vi "AlGaInPAs_prep_run_cont_dil_v00.vi"(2 "Debug Mode":bool, 3 "Elapsed Time(s)":dbl, 4 "State":enum16{"Edit", "Start", "Run", "End", "Idle"}(ring), 5 "Argument List In":string[](array[string])) -> (0 "Status Out":string, 1 "Argument List Out":string[](array[string]))   [LabVIEW 2011]
panel:
  in  "Prep Al":bool caption="Pre-run"
  in  "Run Al":bool caption="Run"
  in  "Al Flow":dbl caption="Al Flow (0-100 sscm)" format="%.2f"
  in  "Ga Tab":enum32{"Page 1", "Page 2"}(tab)
  in  "Prep Ga":bool caption="Pre-run"
  in  "Run Ga":bool caption="Run"
  in  "Ga Flow":dbl caption="Ga Flow (0-100 sscm)" format="%.2f"
  in  "Dilute Ga":bool caption="Dilute"
  in  "GAMFC3":dbl caption="GAMFC3 (0-1000 sccm)"
  out "GAMFC2 set":dbl caption="GAMFC2 (0-100 sscm)" format="%.1f"
  out "GAMFC1 set":dbl caption="GAMFC1 set (0-10 sccm)"
  in  "GAMFC1":dbl caption="GAMFC1 (0-10 sscm)" format="%.2f"
  out "first":bool=TRUE
  out "total time":dbl
  out "is OK?":bool
  out "AsH3?":bool
  out "PH3?":bool
  out "In?":bool
  out "Ga?":bool
  out "Al?":bool
  in  "Prep As":bool caption="Pre-run"
  in  "Prep P":bool caption="Pre-run"
  in  "Prep In":bool caption="Pre-run"
  in  "prep_time":dbl caption="pre-run time (s)"
  in  "Run As":bool caption="Run"
  in  "AsH3 Flow":dbl caption="As Flow (0-10 sccm)" format="%.2f"
  in  "P Flow":dbl caption="P Flow (0-100 sccm)" format="%.2f"
  in  "Run P":bool caption="Run"
  in  "In Flow":dbl caption="In Flow (0-100 sscm)" format="%.2f"
  in  "Run In":bool caption="Run"
  in  "Cancel":bool
  in  "OK":bool
  out "tTotal(s) 2":dbl
  # "Add pre-run time to run time in editor."
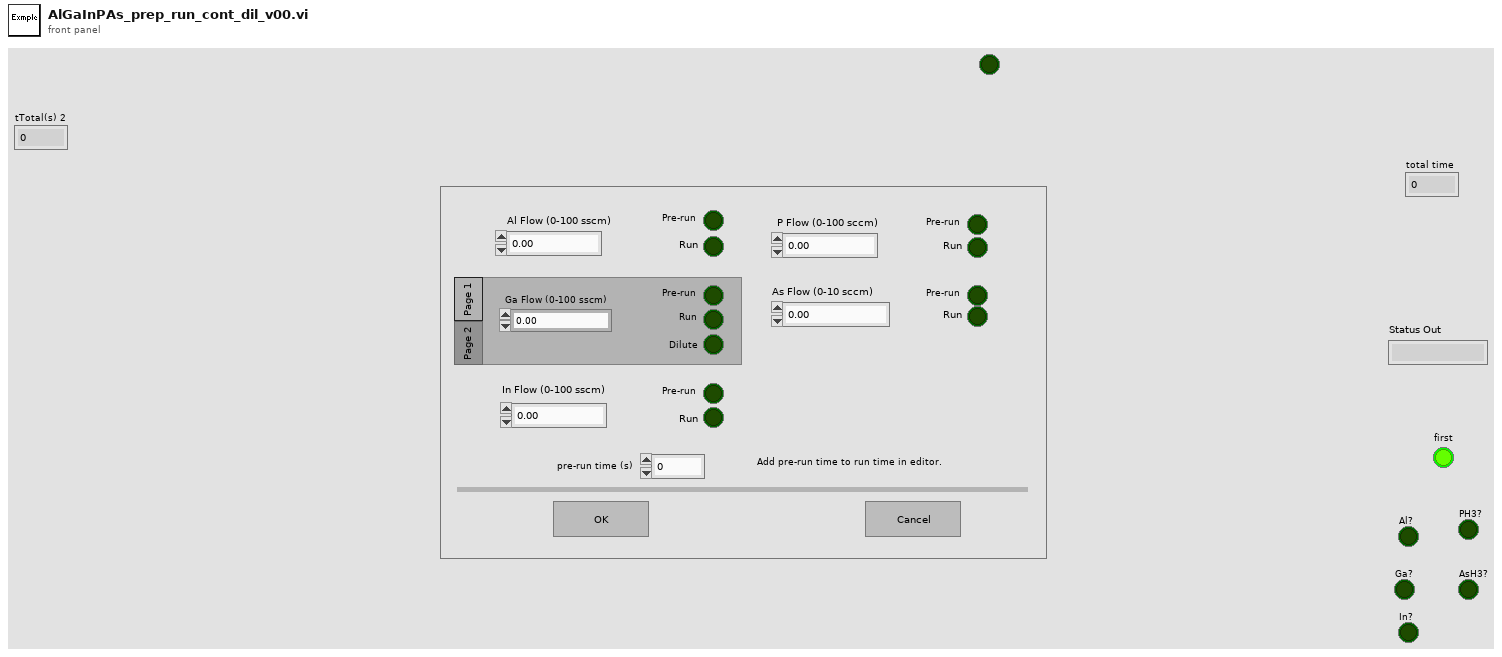
[diagram p1: front panel]
types:
  T1 = enum16{"Discrete", "Continuous", "Instantaneous"}
  T2 = enum32{"Invalid", "Default", "Floating", "Floating/Auto-Hide", "Modal"}
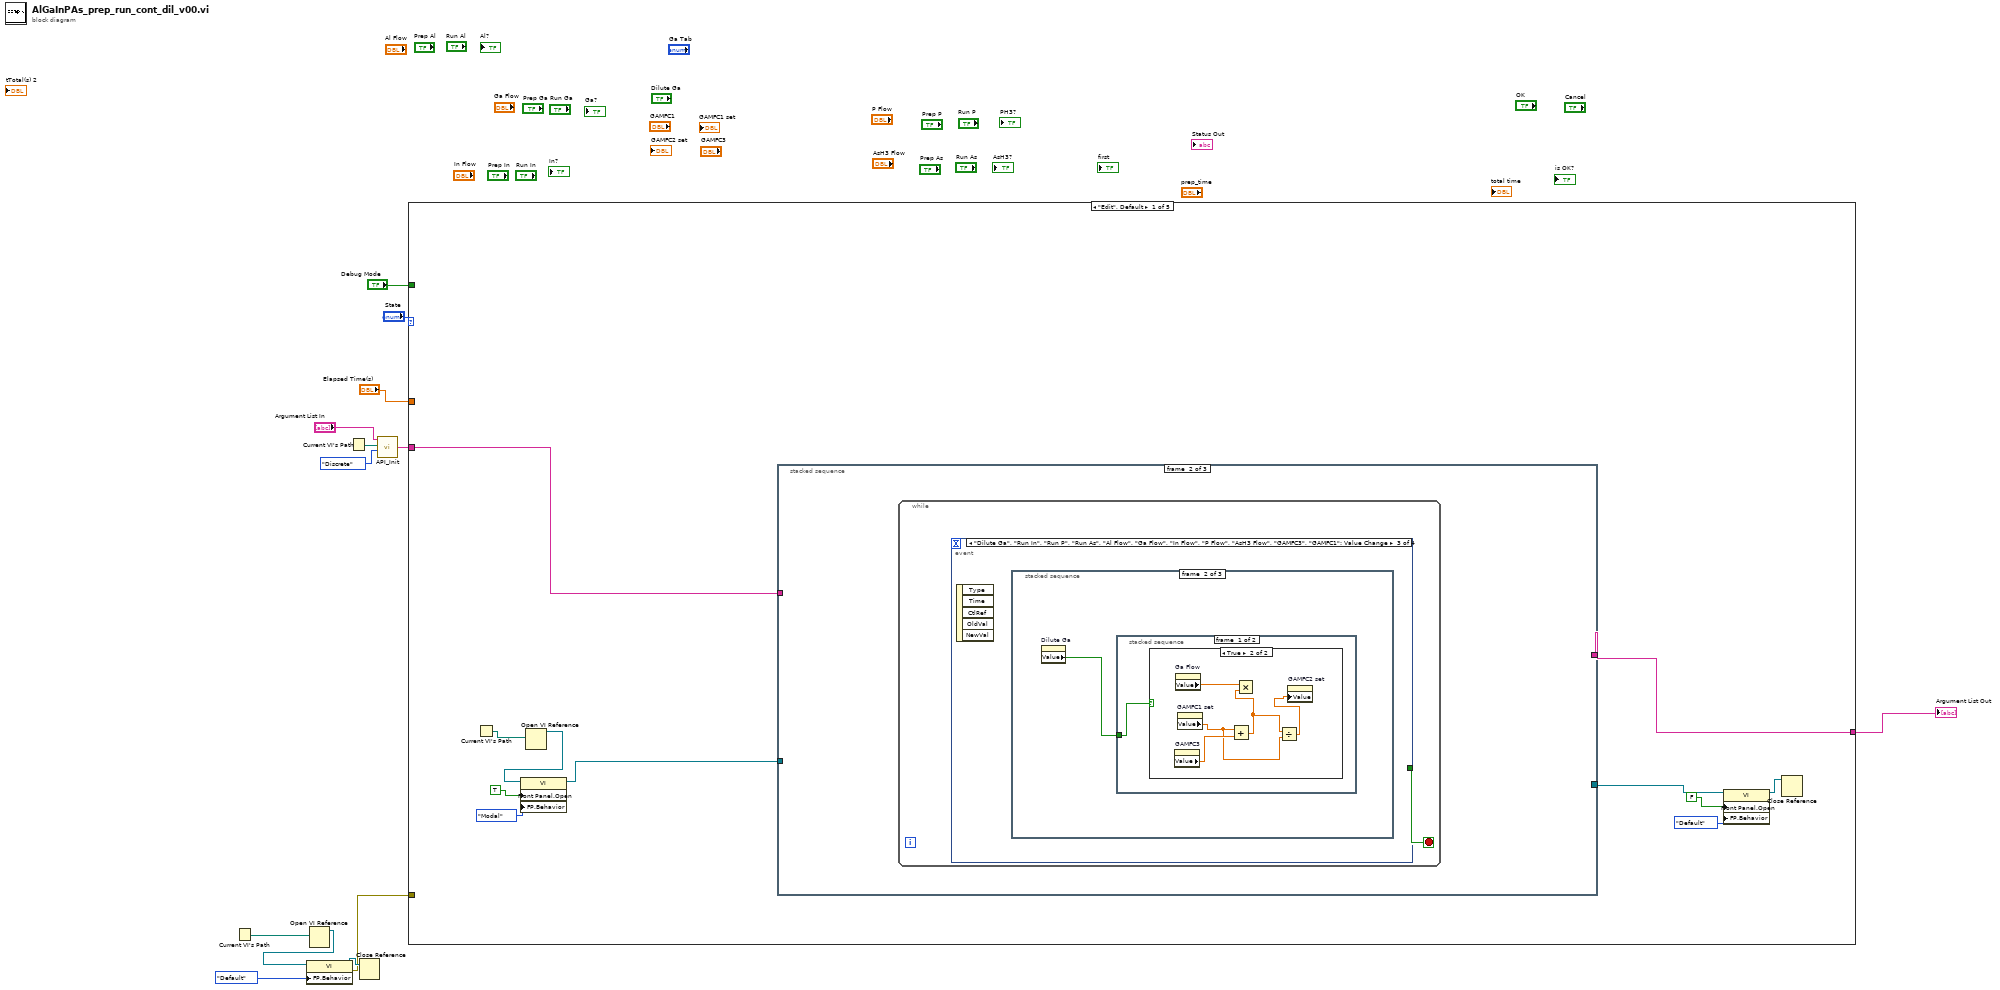
[diagram p0: block diagram]
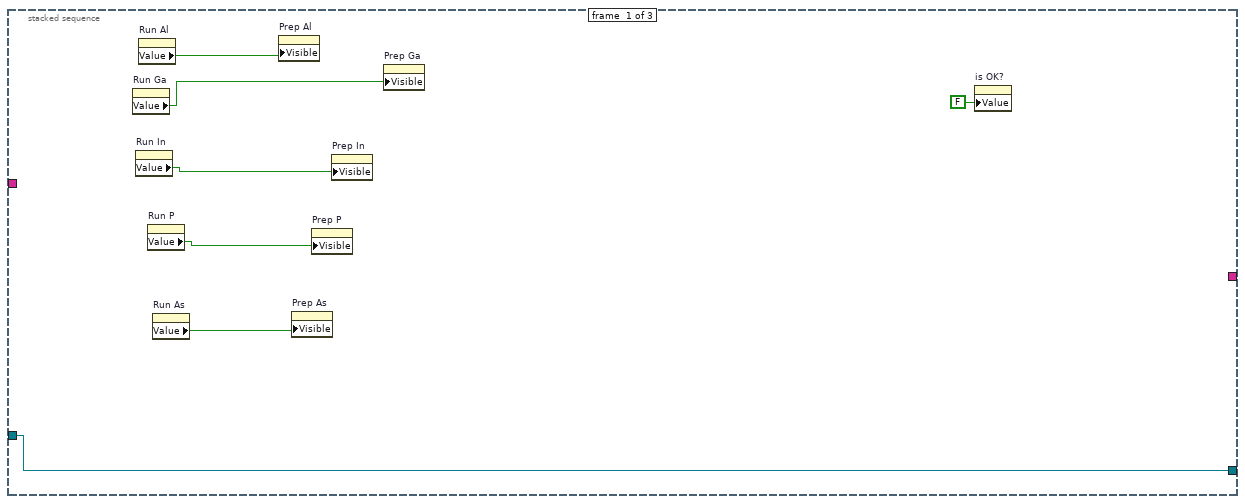
[diagram p2: hidden frame]
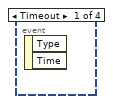
[diagram p3: hidden frame]
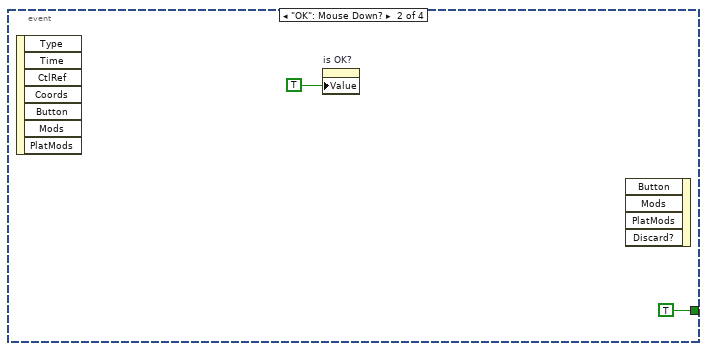
[diagram p4: hidden frame]
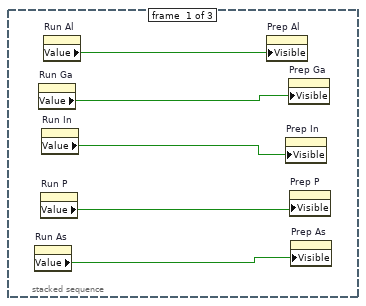
[diagram p5: hidden frame]
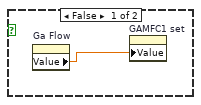
[diagram p6: hidden frame]
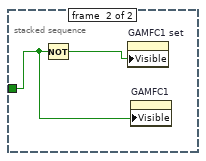
[diagram p7: hidden frame]
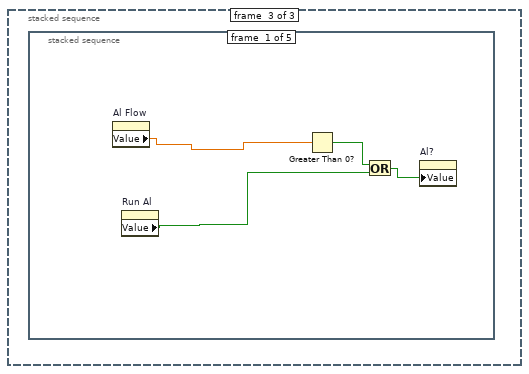
[diagram p8: hidden frame]
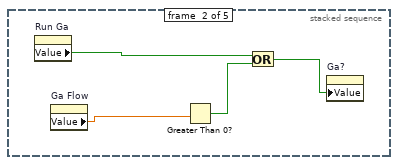
[diagram p9: hidden frame]
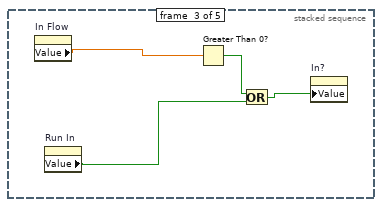
[diagram p10: hidden frame]
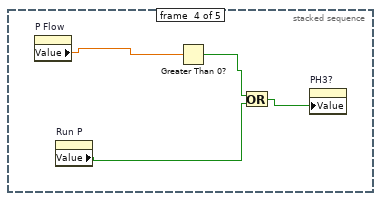
[diagram p11: hidden frame]
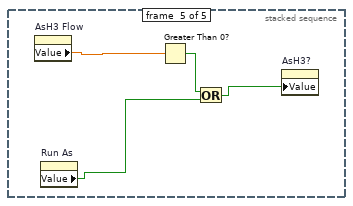
[diagram p12: hidden frame]
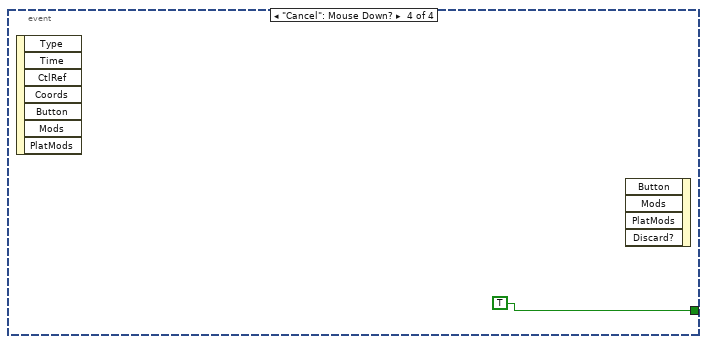
[diagram p13: hidden frame]
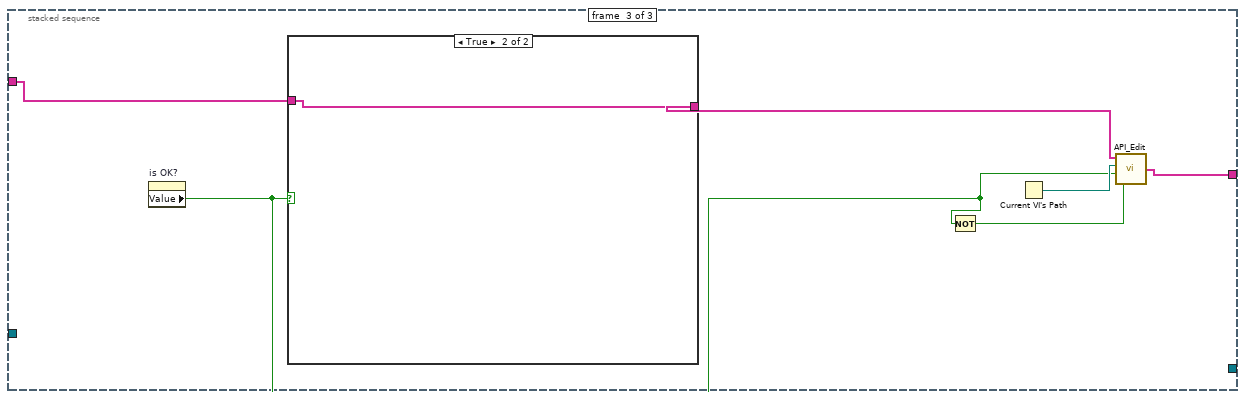
[diagram p14: hidden frame]
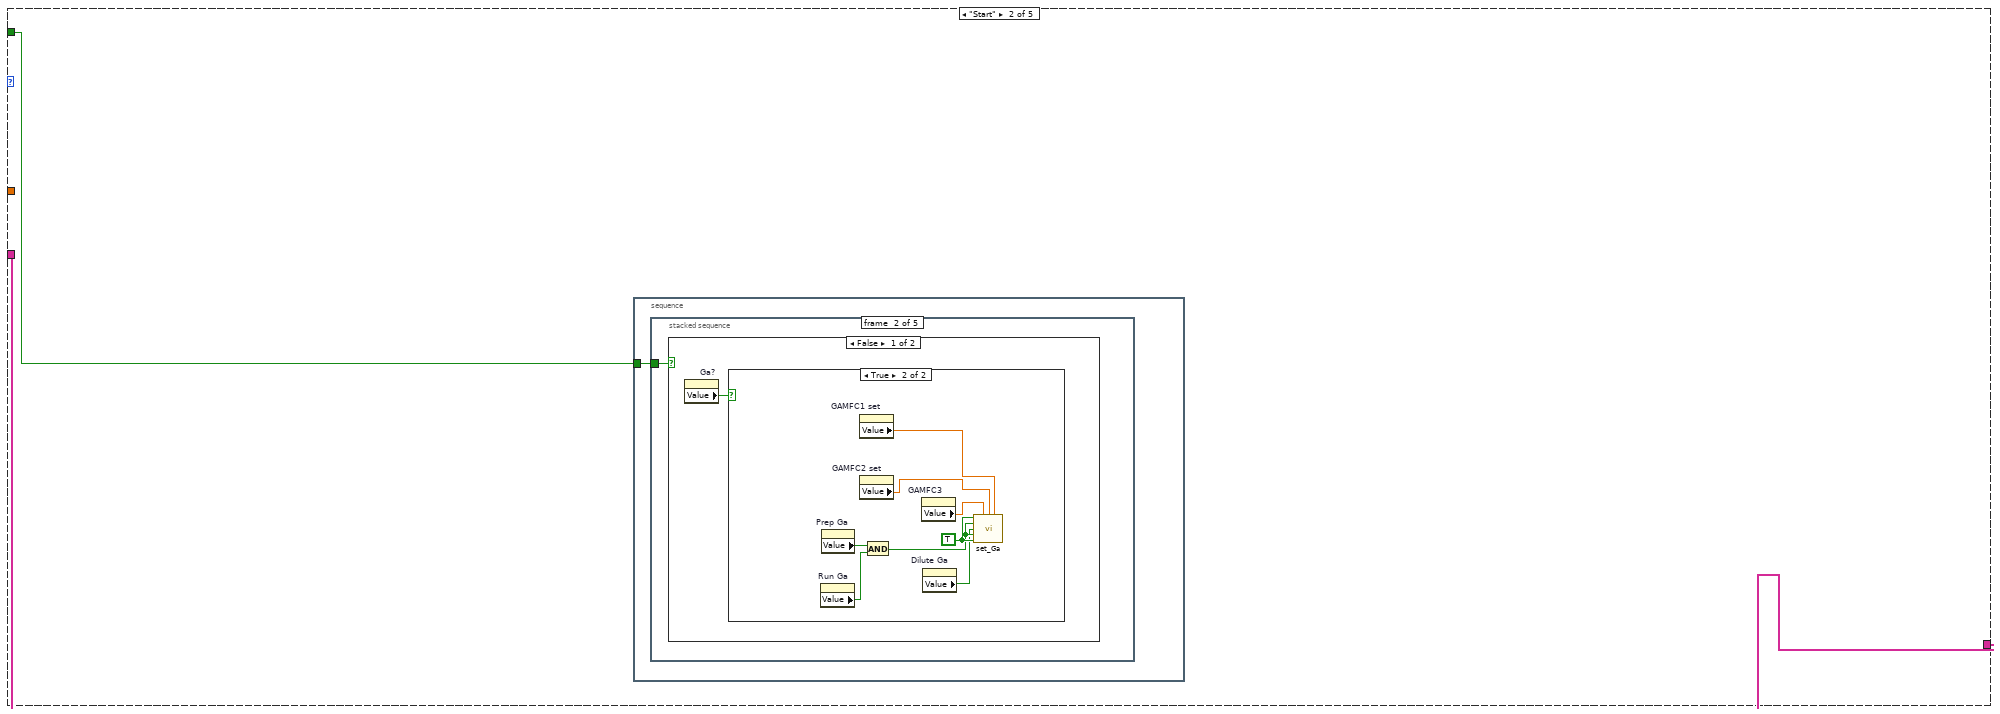
[diagram p16: hidden frame]
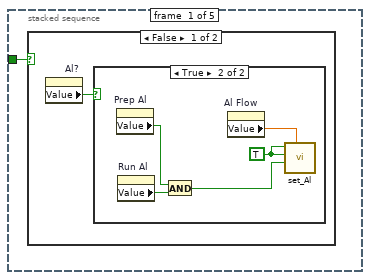
[diagram p17: hidden frame]
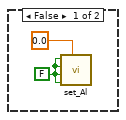
[diagram p18: hidden frame]
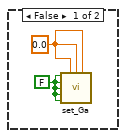
[diagram p20: hidden frame]
diagram:
  n1 = Current VI's Path() -> (path=w9:path)
  n2 = Open VI Reference(vi path=w9) -> (vi reference=w8:refnum<vi>)  [unwired: 1 in, 5 out]
  n3 = property class="VI"(reference=w8, "FP.Behavior"=T2."Default" ("Front Panel Window:Behavior")) -> (reference out=w6:refnum<vi>, error out=w5:errorcluster)  [unwired: 1 in]
  n4 = Current VI's Path() -> (path=w4:path)
  n5 = Close Reference(reference=w6) -> ()  [unwired: 1 in, 1 out]
  n6 = call "API_Init.vi"("API Mode"=T1."Discrete", "VI Path"=w4, "Argument List In"="Argument List In") -> ("Argument List Out"=w1:string[])  [unwired: 1 in]
  n7 = case shown="\"Edit\", Default" "State" {
    tunnel: "Debug Mode" -> [_ w79 w132 _ _]
    tunnel: "Elapsed Time(s)" -> [_ _ w133 _ _]
    tunnel: w1 -> [w15 w80 w135 w224 w225]
    tunnel: [w14 w80 w135 w224 w225] -> w10
    tunnel: w5 -> [_ _ _ _ _]
    frame "Edit", Default {
      n8 = Current VI's Path() -> (path=w20:path)
      n9 = Open VI Reference(vi path=w20) -> (vi reference=w19:refnum<vi>)  [unwired: 1 in, 5 out]
      n10 = property class="VI"(reference=w19, "Front Panel.Open"=TRUE ("Front Panel Window:Open"), "FP.Behavior"=T2."Modal" ("Front Panel Window:Behavior")) -> (reference out=w18:refnum<vi>)  [unwired: 1 in, 1 out]
      n11 = stacked-sequence {
        tunnel: w15 -> [_ _ w74]
        tunnel: w18 -> [w31 _ _]
        tunnel: [w31 _ _] -> w22
        tunnel: [_ _ w72] -> w14
        frame #0 {
          n12 = property on="Run Ga" class="Bool (strict)"() -> ("Value"=w28:bool)  [unwired: 2 in, 2 out]
          n13 = property on="Run In" class="Bool (strict)"() -> ("Value"=w27:bool)  [unwired: 2 in, 2 out]
          n14 = property on="Run Al" class="Bool (strict)"() -> ("Value"=w29:bool)  [unwired: 2 in, 2 out]
          n15 = property on="Run P" class="Bool (strict)"() -> ("Value"=w26:bool)  [unwired: 2 in, 2 out]
          n16 = property on="Run As" class="Bool (strict)"() -> ("Value"=w25:bool)  [unwired: 2 in, 2 out]
          n17 = property on="Prep Al" class="Bool (strict)"("Visible"=w29) -> ()  [unwired: 2 in, 2 out]
          n18 = property on="Prep As" class="Bool (strict)"("Visible"=w25) -> ()  [unwired: 2 in, 2 out]
          n19 = property on="Prep P" class="Bool (strict)"("Visible"=w26) -> ()  [unwired: 2 in, 2 out]
          n20 = property on="Prep In" class="Bool (strict)"("Visible"=w27) -> ()  [unwired: 2 in, 2 out]
          n21 = property on="Prep Ga" class="Bool (strict)"("Visible"=w28) -> ()  [unwired: 2 in, 2 out]
          n22 = property on="is OK?" class="Bool (strict)"("Value"=FALSE ("is OK?")) -> ()  [unwired: 2 in, 2 out]
        }
        frame #1 {
          n23 = while {
            stop <- w32 stop-if-true
            n24 = event shown="[2] \"Dilute Ga\", \"Run In\", \"Run P\", \"Run As\", \"Al Flow\", \"Ga Flow\", \"In Flow\", \"P Flow\", \"AsH3 Flow\", \"GAMFC3\", \"GAMFC1\": Value Change" {
              selector: _ -> [_ _ _ _]
              dyn-events: _ -> [_ _ _ _]
              timeout: _ -> [_ _ _ _]
              tunnel: [_ TRUE _ TRUE] -> w32
              event Timeout {
                n25 = event-data() -> ()  [unwired: 1 in, 2 out]
              }
              event "OK": Mouse Down? {
                n26 = event-data() -> ()  [unwired: 1 in, 7 out]
                n27 = property on="is OK?" class="Bool (strict)"("Value"=TRUE ("is OK?")) -> ()  [unwired: 2 in, 2 out]
                n28 = event-data() -> ()  [unwired: 5 in, 1 out]
              }
              event "Dilute Ga", "Run In", "Run P", "Run As", "Al Flow", "Ga Flow", "In Flow", "P Flow", "AsH3 Flow", "GAMFC3", "GAMFC1": Value Change {
                n29 = event-data() -> ()  [unwired: 1 in, 5 out]
                n30 = stacked-sequence {
                  frame #0 {
                    n31 = property on="Run As" class="Bool (strict)"() -> ("Value"=w35:bool)  [unwired: 2 in, 2 out]
                    n32 = property on="Run Ga" class="Bool (strict)"() -> ("Value"=w38:bool)  [unwired: 2 in, 2 out]
                    n33 = property on="Run P" class="Bool (strict)"() -> ("Value"=w36:bool)  [unwired: 2 in, 2 out]
                    n34 = property on="Run In" class="Bool (strict)"() -> ("Value"=w37:bool)  [unwired: 2 in, 2 out]
                    n35 = property on="Run Al" class="Bool (strict)"() -> ("Value"=w39:bool)  [unwired: 2 in, 2 out]
                    n36 = property on="Prep Al" class="Bool (strict)"("Visible"=w39) -> ()  [unwired: 2 in, 2 out]
                    n37 = property on="Prep In" class="Bool (strict)"("Visible"=w37) -> ()  [unwired: 2 in, 2 out]
                    n38 = property on="Prep Ga" class="Bool (strict)"("Visible"=w38) -> ()  [unwired: 2 in, 2 out]
                    n39 = property on="Prep P" class="Bool (strict)"("Visible"=w36) -> ()  [unwired: 2 in, 2 out]
                    n40 = property on="Prep As" class="Bool (strict)"("Visible"=w35) -> ()  [unwired: 2 in, 2 out]
                  }
                  frame #1 {
                    n41 = property on="Dilute Ga" class="Bool (strict)"() -> ("Value"=w40:bool)  [unwired: 2 in, 2 out]
                    n42 = stacked-sequence {
                      tunnel: w40 -> [w41 w48]
                      frame #0 {
                        n43 = case shown="True" w41 {
                          frame False {
                            n44 = property on="Ga Flow" class="DigNum (strict)"() -> ("Value"=w42:dbl)  [unwired: 2 in, 2 out]
                            n45 = property on="GAMFC1 set" class="DigNum (strict)"("Value"=w42) -> ()  [unwired: 2 in, 2 out]
                          }
                          frame True {
                            n46 = property on="GAMFC3" class="DigNum (strict)"() -> ("Value"=w47:dbl)  [unwired: 2 in, 2 out]
                            n47 = property on="Ga Flow" class="DigNum (strict)"() -> ("Value"=w46:dbl)  [unwired: 2 in, 2 out]
                            n48 = property on="GAMFC1 set" class="DigNum (strict)"() -> ("Value"=w45:dbl)  [unwired: 2 in, 2 out]
                            n49 = Add(x=w45, y=w47) -> (x+y=w44:dbl)
                            n50 = Multiply(x=w46, y=w44) -> ()  [unwired: 1 out]
                            n51 = Divide(x=w44, y=w45) -> (x/y=w43:dbl)
                            n52 = property on="GAMFC2 set" class="DigNum (strict)"("Value"=w43) -> ()  [unwired: 2 in, 2 out]
                          }
                        }
                      }
                      frame #1 {
                        n53 = Not(x=w48) -> (.not. x?=w49:bool)
                        n54 = property on="GAMFC1 set" class="DigNum (strict)"("Visible"=w49) -> ()  [unwired: 2 in, 2 out]
                        n55 = property on="GAMFC1" class="DigNum (strict)"("Visible"=w48) -> ()  [unwired: 2 in, 2 out]
                      }
                    }
                  }
                  frame #2 {
                    n56 = stacked-sequence {
                      frame #0 {
                        n57 = property on="Al Flow" class="DigNum (strict)"() -> ("Value"=w52:dbl)  [unwired: 2 in, 2 out]
                        n58 = property on="Run Al" class="Bool (strict)"() -> ("Value"=w51:bool)  [unwired: 2 in, 2 out]
                        n59 = Greater Than 0?(x=w52) -> (x > 0?=w53:bool)
                        n60 = Or(x=w53, y=w51) -> (x .or. y?=w50:bool)
                        n61 = property on="Al?" class="Bool (strict)"("Value"=w50) -> ()  [unwired: 2 in, 2 out]
                      }
                      frame #1 {
                        n62 = property on="Run Ga" class="Bool (strict)"() -> ("Value"=w55:bool)  [unwired: 2 in, 2 out]
                        n63 = property on="Ga Flow" class="DigNum (strict)"() -> ("Value"=w56:dbl)  [unwired: 2 in, 2 out]
                        n64 = Greater Than 0?(x=w56) -> (x > 0?=w57:bool)
                        n65 = Or(x=w55, y=w57) -> (x .or. y?=w54:bool)
                        n66 = property on="Ga?" class="Bool (strict)"("Value"=w54) -> ()  [unwired: 2 in, 2 out]
                      }
                      frame #2 {
                        n67 = property on="In Flow" class="DigNum (strict)"() -> ("Value"=w59:dbl)  [unwired: 2 in, 2 out]
                        n68 = property on="Run In" class="Bool (strict)"() -> ("Value"=w60:bool)  [unwired: 2 in, 2 out]
                        n69 = Greater Than 0?(x=w59) -> (x > 0?=w61:bool)
                        n70 = Or(x=w61, y=w60) -> (x .or. y?=w58:bool)
                        n71 = property on="In?" class="Bool (strict)"("Value"=w58) -> ()  [unwired: 2 in, 2 out]
                      }
                      frame #3 {
                        n72 = property on="P Flow" class="DigNum (strict)"() -> ("Value"=w64:dbl)  [unwired: 2 in, 2 out]
                        n73 = property on="Run P" class="Bool (strict)"() -> ("Value"=w63:bool)  [unwired: 2 in, 2 out]
                        n74 = Greater Than 0?(x=w64) -> (x > 0?=w65:bool)
                        n75 = Or(x=w65, y=w63) -> (x .or. y?=w62:bool)
                        n76 = property on="PH3?" class="Bool (strict)"("Value"=w62) -> ()  [unwired: 2 in, 2 out]
                      }
                      frame #4 {
                        n77 = property on="AsH3 Flow" class="DigNum (strict)"() -> ("Value"=w68:dbl)  [unwired: 2 in, 2 out]
                        n78 = property on="Run As" class="Bool (strict)"() -> ("Value"=w67:bool)  [unwired: 2 in, 2 out]
                        n79 = Greater Than 0?(x=w68) -> (x > 0?=w69:bool)
                        n80 = Or(x=w69, y=w67) -> (x .or. y?=w66:bool)
                        n81 = property on="AsH3?" class="Bool (strict)"("Value"=w66) -> ()  [unwired: 2 in, 2 out]
                      }
                    }
                  }
                }
              }
              event "Cancel": Mouse Down? {
                n82 = event-data() -> ()  [unwired: 1 in, 7 out]
                n83 = event-data() -> ()  [unwired: 5 in, 1 out]
              }
            }
          }
        }
        frame #2 {
          n84 = property on="is OK?" class="Bool (strict)"() -> ("Value"=w71:bool)  [unwired: 2 in, 2 out]
          n85 = case shown="True" w71 {
            tunnel: w74 -> [w77 w78]
            tunnel: [w77 w78] -> w73
            frame False {
            }
            frame True {
            }
          }
          n86 = Not(x=w71) -> (.not. x?=w76:bool)
          n87 = Current VI's Path() -> (path=w75:path)
          n88 = call "API_Edit.vi"("Cancel"=w76, "OK"=w71, "VI Path"=w75, "Argument List In"=w73) -> ("Argument List Out"=w72:string[])
        }
      }
      n89 = property class="VI"(reference=w22, "Front Panel.Open"=FALSE ("Front Panel Window:Open"), "FP.Behavior"=T2."Default" ("Front Panel Window:Behavior")) -> (reference out=w23:refnum<vi>)  [unwired: 1 in, 1 out]
      n90 = Close Reference(reference=w23) -> ()  [unwired: 1 in, 1 out]
    }
    frame "Start" {
      n91 = stacked-sequence {
        tunnel: w79 -> [w81]
        frame #0 {
          n92 = stacked-sequence {
            tunnel: w81 -> [w82 w91 w103 w112 w121]
            frame #0 {
              n93 = case shown="False" w82 {
                frame False {
                  n94 = property on="Al?" class="Bool (strict)"() -> ("Value"=w83:bool)  [unwired: 2 in, 2 out]
                  n95 = case shown="True" w83 {
                    frame False {
                      w84 = FALSE ("Al Active")
                      n96 = call "set_Al.vi"("Aluminum Flow"=0.0, "Al Remote"=w84, "Al Run"=w84, "Al Bubbler"=w84, "Al Active"=w84) -> ()  [unwired: 5 out]
                    }
                    frame True {
                      w90 = TRUE ("Al Active")
                      n97 = property on="Prep Al" class="Bool (strict)"() -> ("Value"=w88:bool)  [unwired: 2 in, 2 out]
                      n98 = property on="Run Al" class="Bool (strict)"() -> ("Value"=w87:bool)  [unwired: 2 in, 2 out]
                      n99 = And(x=w88, y=w87) -> (x .and. y?=w86:bool)
                      n100 = property on="Al Flow" class="DigNum (strict)"() -> ("Value"=w89:dbl)  [unwired: 2 in, 2 out]
                      n101 = call "set_Al.vi"("Aluminum Flow"=w89, "Al Run"=w86, "Al Bubbler"=w90, "Al Active"=w90) -> ()  [unwired: 1 in, 5 out]
                    }
                  }
                }
                frame True {
                }
              }
            }
            frame #1 {
              n102 = case shown="False" w91 {
                frame False {
                  n103 = property on="Ga?" class="Bool (strict)"() -> ("Value"=w92:bool)  [unwired: 2 in, 2 out]
                  n104 = case shown="True" w92 {
                    frame False {
                      w94 = FALSE ("Ga Active")
                      w93 = 0.0 ("Ga Flow 1")
                      n105 = call "set_Ga.vi"("Ga Active"=w94, "Ga Flow 3"=w93, "Ga Flow 2"=w93, "Ga Flow 1"=w93, "Ga Bubbler"=w94, "Ga H2 Dilute"=w94, "Ga Run"=w94, "Ga Remote"=w94) -> ()  [unwired: 8 out]
                    }
                    frame True {
                      w100 = TRUE ("Ga Active")
                      n106 = property on="Run Ga" class="Bool (strict)"() -> ("Value"=w101:bool)  [unwired: 2 in, 2 out]
                      n107 = property on="Prep Ga" class="Bool (strict)"() -> ("Value"=w102:bool)  [unwired: 2 in, 2 out]
                      n108 = property on="GAMFC1 set" class="DigNum (strict)"() -> ("Value"=w98:dbl)  [unwired: 2 in, 2 out]
                      n109 = property on="GAMFC2 set" class="DigNum (strict)"() -> ("Value"=w97:dbl)  [unwired: 2 in, 2 out]
                      n110 = And(x=w102, y=w101) -> (x .and. y?=w99:bool)
                      n111 = property on="GAMFC3" class="DigNum (strict)"() -> ("Value"=w96:dbl)  [unwired: 2 in, 2 out]
                      n112 = property on="Dilute Ga" class="Bool (strict)"() -> ("Value"=w95:bool)  [unwired: 2 in, 2 out]
                      n113 = call "set_Ga.vi"("Ga Active"=w100, "Ga Flow 3"=w96, "Ga Flow 2"=w97, "Ga Flow 1"=w98, "Ga Bubbler"=w99, "Ga H2 Dilute"=w95, "Ga Run"=w99, "Ga Remote"=w100) -> ()  [unwired: 8 in]
                    }
                  }
                }
                frame True {
                }
              }
            }
            frame #2 {
              n114 = case shown="False" w103 {
                frame False {
                  n115 = property on="In?" class="Bool (strict)"() -> ("Value"=w104:bool)  [unwired: 2 in, 2 out]
                  n116 = case shown="True" w104 {
                    frame False {
                      w106 = FALSE ("In Remote")
                      n117 = call "set_In.vi"("Indium Flow"=0.0, "In Remote"=w106, "In Run"=w106, "In Bubbler"=w106, "In Active"=w106) -> ()  [unwired: 5 out]
                    }
                    frame True {
                      w111 = TRUE ("In Run")
                      n118 = property on="Prep In" class="Bool (strict)"() -> ("Value"=w109:bool)  [unwired: 2 in, 2 out]
                      n119 = property on="Run In" class="Bool (strict)"() -> ("Value"=w108:bool)  [unwired: 2 in, 2 out]
                      n120 = And(x=w109, y=w108) -> (x .and. y?=w107:bool)
                      n121 = property on="In Flow" class="DigNum (strict)"() -> ("Value"=w110:dbl)  [unwired: 2 in, 2 out]
                      n122 = call "set_In.vi"("Indium Flow"=w110, "In Run"=w107, "In Bubbler"=w111, "In Active"=w111) -> ()  [unwired: 1 in, 5 out]
                    }
                  }
                }
                frame True {
                }
              }
            }
            frame #3 {
              n123 = case shown="False" w112 {
                frame False {
                  n124 = property on="PH3?" class="Bool (strict)"() -> ("Value"=w113:bool)  [unwired: 2 in, 2 out]
                  n125 = case shown="True" w113 {
                    frame False {
                      w114 = FALSE ("P_Gas Active")
                      n126 = call "set_P_gas.vi"("P_Gas Active"=w114, "P_Gas Flow"=0.0, "P_Gas In"=w114, "P_Gas H2 In"=w114, "P_Gas Run"=w114, "P_Gas Remote"=w114) -> ()  [unwired: 10 out]
                    }
                    frame True {
                      w120 = TRUE ("P_Gas Active")
                      n127 = property on="Prep P" class="Bool (strict)"() -> ("Value"=w118:bool)  [unwired: 2 in, 2 out]
                      n128 = property on="Run P" class="Bool (strict)"() -> ("Value"=w117:bool)  [unwired: 2 in, 2 out]
                      n129 = And(x=w118, y=w117) -> (x .and. y?=w116:bool)
                      n130 = property on="P Flow" class="DigNum (strict)"() -> ("Value"=w119:dbl)  [unwired: 2 in, 2 out]
                      n131 = call "set_P_gas.vi"("P_Gas Active"=w120, "P_Gas Flow"=w119, "P_Gas In"=w120, "P_Gas Run"=w116) -> ()  [unwired: 2 in, 10 out]
                    }
                  }
                }
                frame True {
                }
              }
            }
            frame #4 {
              n132 = case shown="False" w121 {
                frame False {
                  n133 = property on="AsH3?" class="Bool (strict)"() -> ("Value"=w122:bool)  [unwired: 2 in, 2 out]
                  n134 = case shown="True" w122 {
                    frame False {
                      w123 = FALSE ("As_Gas Active")
                      n135 = call "set_As_gas.vi"("As_Gas Active"=w123, "As_Gas Flow"=0.0, "As_Gas In"=w123, "As_Gas H2"=w123, "As_Gas Run"=w123, "As_Gas Remote"=w123) -> ()  [unwired: 10 in]
                    }
                    frame True {
                      w129 = TRUE ("As_Gas Active")
                      n136 = property on="Prep As" class="Bool (strict)"() -> ("Value"=w126:bool)  [unwired: 2 in, 2 out]
                      n137 = property on="Run As" class="Bool (strict)"() -> ("Value"=w127:bool)  [unwired: 2 in, 2 out]
                      n138 = And(x=w126, y=w127) -> (x .and. y?=w125:bool)
                      n139 = property on="AsH3 Flow" class="DigNum (strict)"() -> ("Value"=w128:dbl)  [unwired: 2 in, 2 out]
                      n140 = call "set_As_gas.vi"("As_Gas Active"=w129, "As_Gas Flow"=w128, "As_Gas In"=w129, "As_Gas Run"=w125) -> ()  [unwired: 12 in]
                    }
                  }
                }
                frame True {
                }
              }
            }
          }
        }
      }
    }
    frame "Run" {
      n141 = property on="prep_time" class="DigNum (strict)"() -> ("Value"=w134:dbl)  [unwired: 2 in, 2 out]
      n142 = Greater Or Equal?(x=w133, y=w134) -> (x >= y?=w131:bool)
      n143 = Not(x=w131) -> (.not. x?=w130:bool)
      n144 = stacked-sequence {
        tunnel: w130 -> [w137 w141 w150 w159 w168 w177]
        frame #0 {
          n145 = case shown="True" w137 {
            tunnel: ["run: " "pre-run: "] -> w136
            frame False {
            }
            frame True {
            }
          }
          n146 = property on="Status Out" class="Str"("Value"=w136) -> ()  [unwired: 2 in, 2 out]
        }
        frame #1 {
          n147 = property on="Status Out" class="Str"() -> ("Value"=w147:string)  [unwired: 2 in, 2 out]
          n148 = property on="Al?" class="Bool (strict)"() -> ("Value"=w148:bool)  [unwired: 2 in, 2 out]
          n149 = property on="Run Al" class="Bool (strict)"() -> ("Value"=w140:bool)  [unwired: 2 in, 2 out]
          n150 = property on="Prep Al" class="Bool (strict)"() -> ("Value"=w142:bool)  [unwired: 2 in, 2 out]
          n151 = call "flow_strings.vi"("string in"=w147, "is first in?"=TRUE, "use source?"=w148, "name"="Al", "run source?"=w140, "prep source?"=w142, "is prep?"=w141) -> ("string out"=w146:string, "is first out?"=w145:bool)
          n152 = property on="Status Out" class="Str"("Value"=w146) -> ()  [unwired: 2 in, 2 out]
          n153 = property on="first" class="Bool (strict)"("Value"=w145) -> ()  [unwired: 2 in, 2 out]
        }
        frame #2 {
          n154 = property on="first" class="Bool (strict)"() -> ("Value"=w153:bool)  [unwired: 2 in, 2 out]
          n155 = property on="Status Out" class="Str"() -> ("Value"=w156:string)  [unwired: 2 in, 2 out]
          n156 = property on="Ga?" class="Bool (strict)"() -> ("Value"=w154:bool)  [unwired: 2 in, 2 out]
          n157 = property on="Run Ga" class="Bool (strict)"() -> ("Value"=w149:bool)  [unwired: 2 in, 2 out]
          n158 = property on="Prep Ga" class="Bool (strict)"() -> ("Value"=w151:bool)  [unwired: 2 in, 2 out]
          n159 = call "flow_strings.vi"("string in"=w156, "is first in?"=w153, "use source?"=w154, "name"="Ga", "run source?"=w149, "prep source?"=w151, "is prep?"=w150) -> ("string out"=w157:string, "is first out?"=w152:bool)
          n160 = property on="Status Out" class="Str"("Value"=w157) -> ()  [unwired: 2 in, 2 out]
          n161 = property on="first" class="Bool (strict)"("Value"=w152) -> ()  [unwired: 2 in, 2 out]
        }
        frame #3 {
          n162 = property on="first" class="Bool (strict)"() -> ("Value"=w163:bool)  [unwired: 2 in, 2 out]
          n163 = property on="Status Out" class="Str"() -> ("Value"=w165:string)  [unwired: 2 in, 2 out]
          n164 = property on="In?" class="Bool (strict)"() -> ("Value"=w166:bool)  [unwired: 2 in, 2 out]
          n165 = property on="Run In" class="Bool (strict)"() -> ("Value"=w158:bool)  [unwired: 2 in, 2 out]
          n166 = property on="Prep In" class="Bool (strict)"() -> ("Value"=w160:bool)  [unwired: 2 in, 2 out]
          n167 = call "flow_strings.vi"("string in"=w165, "is first in?"=w163, "use source?"=w166, "name"="In", "run source?"=w158, "prep source?"=w160, "is prep?"=w159) -> ("string out"=w162:string, "is first out?"=w161:bool)
          n168 = property on="Status Out" class="Str"("Value"=w162) -> ()  [unwired: 2 in, 2 out]
          n169 = property on="first" class="Bool (strict)"("Value"=w161) -> ()  [unwired: 2 in, 2 out]
        }
        frame #4 {
          n170 = property on="first" class="Bool (strict)"() -> ("Value"=w171:bool)  [unwired: 2 in, 2 out]
          n171 = property on="Status Out" class="Str"() -> ("Value"=w173:string)  [unwired: 2 in, 2 out]
          n172 = property on="PH3?" class="Bool (strict)"() -> ("Value"=w174:bool)  [unwired: 2 in, 2 out]
          n173 = property on="Run P" class="Bool (strict)"() -> ("Value"=w167:bool)  [unwired: 2 in, 2 out]
          n174 = property on="Prep P" class="Bool (strict)"() -> ("Value"=w169:bool)  [unwired: 2 in, 2 out]
          n175 = call "flow_strings.vi"("string in"=w173, "is first in?"=w171, "use source?"=w174, "name"="P", "run source?"=w167, "prep source?"=w169, "is prep?"=w168) -> ("string out"=w172:string, "is first out?"=w170:bool)
          n176 = property on="Status Out" class="Str"("Value"=w172) -> ()  [unwired: 2 in, 2 out]
          n177 = property on="first" class="Bool (strict)"("Value"=w170) -> ()  [unwired: 2 in, 2 out]
        }
        frame #5 {
          n178 = property on="first" class="Bool (strict)"() -> ("Value"=w180:bool)  [unwired: 2 in, 2 out]
          n179 = property on="Status Out" class="Str"() -> ("Value"=w182:string)  [unwired: 2 in, 2 out]
          n180 = property on="AsH3?" class="Bool (strict)"() -> ("Value"=w183:bool)  [unwired: 2 in, 2 out]
          n181 = property on="Run As" class="Bool (strict)"() -> ("Value"=w176:bool)  [unwired: 2 in, 2 out]
          n182 = property on="Prep As" class="Bool (strict)"() -> ("Value"=w178:bool)  [unwired: 2 in, 2 out]
          n183 = call "flow_strings.vi"("string in"=w182, "is first in?"=w180, "use source?"=w183, "name"="As", "run source?"=w176, "prep source?"=w178, "is prep?"=w177) -> ("string out"=w179:string, "is first out?"=w181:bool)
          n184 = property on="Status Out" class="Str"("Value"=w179) -> ()  [unwired: 2 in, 2 out]
          n185 = property on="first" class="Bool (strict)"("Value"=w181) -> ()  [unwired: 2 in, 2 out]
        }
      }
      n186 = case shown="True" w131 {
        tunnel: w132 -> [_ w185]
        frame False {
        }
        frame True {
          n187 = stacked-sequence {
            tunnel: w185 -> [w186 w193 w203 w210 w217]
            frame #0 {
              n188 = case shown="True" w186 {
                frame False {
                  n189 = property on="Al?" class="Bool (strict)"() -> ("Value"=w187:bool)  [unwired: 2 in, 2 out]
                  n190 = case shown="True" w187 {
                    frame False {
                      w188 = FALSE ("Al Active")
                      n191 = call "set_Al.vi"("Aluminum Flow"=0.0, "Al Remote"=w188, "Al Run"=w188, "Al Bubbler"=w188, "Al Active"=w188) -> ()  [unwired: 5 out]
                    }
                    frame True {
                      w192 = TRUE ("Al Active")
                      n192 = property on="Al Flow" class="DigNum (strict)"() -> ("Value"=w191:dbl)  [unwired: 2 in, 2 out]
                      n193 = property on="Run Al" class="Bool (strict)"() -> ("Value"=w190:bool)  [unwired: 2 in, 2 out]
                      n194 = call "set_Al.vi"("Aluminum Flow"=w191, "Al Run"=w190, "Al Bubbler"=w192, "Al Active"=w192) -> ()  [unwired: 1 in, 5 out]
                    }
                  }
                }
                frame True {
                }
              }
            }
            frame #1 {
              n195 = case shown="False" w193 {
                frame False {
                  n196 = property on="Ga?" class="Bool (strict)"() -> ("Value"=w194:bool)  [unwired: 2 in, 2 out]
                  n197 = case shown="True" w194 {
                    frame False {
                      w196 = FALSE ("Ga Active")
                      w195 = 0.0 ("Ga Flow 1")
                      n198 = call "set_Ga.vi"("Ga Active"=w196, "Ga Flow 3"=w195, "Ga Flow 2"=w195, "Ga Flow 1"=w195, "Ga Bubbler"=w196, "Ga H2 Dilute"=w196, "Ga Run"=w196, "Ga Remote"=w196) -> ()  [unwired: 8 out]
                    }
                    frame True {
                      w199 = TRUE ("Ga Active")
                      n199 = property on="GAMFC1 set" class="DigNum (strict)"() -> ("Value"=w197:dbl)  [unwired: 2 in, 2 out]
                      n200 = property on="Dilute Ga" class="Bool (strict)"() -> ("Value"=w198:bool)  [unwired: 2 in, 2 out]
                      n201 = property on="Run Ga" class="Bool (strict)"() -> ("Value"=w200:bool)  [unwired: 2 in, 2 out]
                      n202 = property on="GAMFC2 set" class="DigNum (strict)"() -> ("Value"=w201:dbl)  [unwired: 2 in, 2 out]
                      n203 = property on="GAMFC3" class="DigNum (strict)"() -> ("Value"=w202:dbl)  [unwired: 2 in, 2 out]
                      n204 = call "set_Ga.vi"("Ga Active"=w199, "Ga Flow 3"=w202, "Ga Flow 2"=w201, "Ga Flow 1"=w197, "Ga Bubbler"=w199, "Ga H2 Dilute"=w198, "Ga Run"=w200, "Ga Remote"=w199) -> ()  [unwired: 8 in]
                    }
                  }
                }
                frame True {
                }
              }
            }
            frame #2 {
              n205 = case shown="False" w203 {
                frame False {
                  n206 = property on="In?" class="Bool (strict)"() -> ("Value"=w204:bool)  [unwired: 2 in, 2 out]
                  n207 = case shown="True" w204 {
                    frame False {
                      w206 = FALSE ("In Remote")
                      n208 = call "set_In.vi"("Indium Flow"=0.0, "In Remote"=w206, "In Run"=w206, "In Bubbler"=w206, "In Active"=w206) -> ()  [unwired: 5 out]
                    }
                    frame True {
                      w209 = TRUE ("In Run")
                      n209 = property on="Run In" class="Bool (strict)"() -> ("Value"=w207:bool)  [unwired: 2 in, 2 out]
                      n210 = property on="In Flow" class="DigNum (strict)"() -> ("Value"=w208:dbl)  [unwired: 2 in, 2 out]
                      n211 = call "set_In.vi"("Indium Flow"=w208, "In Run"=w207, "In Bubbler"=w209, "In Active"=w209) -> ()  [unwired: 1 in, 5 out]
                    }
                  }
                }
                frame True {
                }
              }
            }
            frame #3 {
              n212 = case shown="False" w210 {
                frame False {
                  n213 = property on="PH3?" class="Bool (strict)"() -> ("Value"=w211:bool)  [unwired: 2 in, 2 out]
                  n214 = case shown="False" w211 {
                    frame False {
                      w212 = FALSE ("P_Gas Active")
                      n215 = call "set_P_gas.vi"("P_Gas Active"=w212, "P_Gas Flow"=0.0, "P_Gas In"=w212, "P_Gas H2 In"=w212, "P_Gas Run"=w212, "P_Gas Remote"=w212) -> ()  [unwired: 10 out]
                    }
                    frame True {
                      w216 = TRUE ("P_Gas Active")
                      n216 = property on="P Flow" class="DigNum (strict)"() -> ("Value"=w215:dbl)  [unwired: 2 in, 2 out]
                      n217 = property on="Run P" class="Bool (strict)"() -> ("Value"=w214:bool)  [unwired: 2 in, 2 out]
                      n218 = call "set_P_gas.vi"("P_Gas Active"=w216, "P_Gas Flow"=w215, "P_Gas In"=w216, "P_Gas Run"=w214) -> ()  [unwired: 2 in, 10 out]
                    }
                  }
                }
                frame True {
                }
              }
            }
            frame #4 {
              n219 = case shown="False" w217 {
                frame False {
                  n220 = property on="AsH3?" class="Bool (strict)"() -> ("Value"=w218:bool)  [unwired: 2 in, 2 out]
                  n221 = case shown="True" w218 {
                    frame False {
                      w219 = FALSE ("As_Gas Active")
                      n222 = call "set_As_gas.vi"("As_Gas Active"=w219, "As_Gas Flow"=0.0, "As_Gas In"=w219, "As_Gas H2"=w219, "As_Gas Run"=w219, "As_Gas Remote"=w219) -> ()  [unwired: 10 in]
                    }
                    frame True {
                      w222 = TRUE ("As_Gas Active")
                      n223 = property on="Run As" class="Bool (strict)"() -> ("Value"=w221:bool)  [unwired: 2 in, 2 out]
                      n224 = property on="AsH3 Flow" class="DigNum (strict)"() -> ("Value"=w223:dbl)  [unwired: 2 in, 2 out]
                      n225 = call "set_As_gas.vi"("As_Gas Active"=w222, "As_Gas Flow"=w223, "As_Gas In"=w222, "As_Gas Run"=w221) -> ()  [unwired: 12 in]
                    }
                  }
                }
                frame True {
                }
              }
            }
          }
        }
      }
    }
    frame "End" {
    }
    frame "Idle" {
    }
  }
  "Argument List Out" <- w10
